vi "sv_Check dt.vi"(6 "check dt continuity (F)":bool, 8 "error in":errorcluster, 10 "dt":dbl) -> (0 "error out":errorcluster, 2 "dt changed":bool)   [LabVIEW 2017, in "SoundVib_Distortion.lvlib"]
uses:
  <vilib>/addons/Sound and Vibration/svt_Distortion/SoundVib_Distortion.lvlib
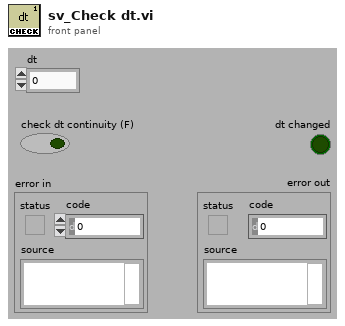
[diagram p1: front panel]
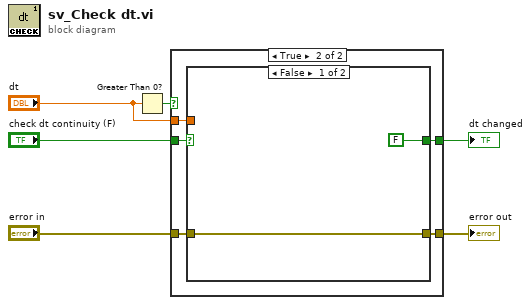
[diagram p0: block diagram]
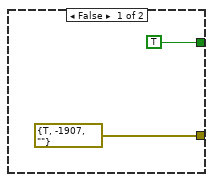
[diagram p2: hidden frame]
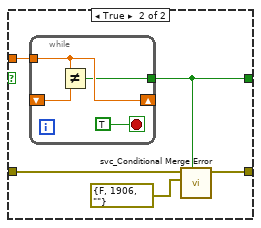
[diagram p3: hidden frame]
diagram:
  n1 = Greater Than 0?(x="dt") -> (x > 0?=w1:bool)
  n2 = case shown="True" w1 {
    tunnel: "dt" -> [_ w13]
    tunnel: "error in" -> [_ w12]
    tunnel: [errorcluster {"status"=TRUE, "code"=-1907, "source"=""} ("error IO") w11] -> w3
    tunnel: [TRUE w10] -> w4
    tunnel: "check dt continuity (F)" -> [_ w9]
    frame False {
    }
    frame True {
      n3 = case shown="False" w9 {
        tunnel: w13 -> [_ w20]
        tunnel: w12 -> [w15 w19]
        tunnel: [w15 w18] -> w11
        tunnel: [FALSE w17] -> w10
        frame False {
        }
        frame True {
          n4 = while {
            tunnel: [w21] -> w17
            tunnel: w20 -> [w23]
            shift-left: _ -> [w22]
            shift-right: [w23] -> _
            stop <- TRUE stop-if-true
            n5 = Not Equal?(x=w23, y=w22) -> (x != y?=w21:bool)
          }
          n6 = call <vilib>:"svc_Conditional Merge Error.vi"("merge"=w17, "new error"=errorcluster {"status"=FALSE, "code"=1906, "source"=""} ("error IO"), "error in (no error)"=w19) -> ("error out"=w18:errorcluster)  [unwired: 8 in]
        }
      }
    }
  }
  "dt changed" <- w4
  "error out" <- w3
